vi "Reset Timer.vi"(8 "error in (no error)":errorcluster, 10 "Timer No. (0: All timer number )":string="0", 11 "VISA resource name":refnum<visa-resource-name>) -> (0 "error out":errorcluster, 3 "VISA resource name out":refnum<visa-resource-name>)   [LabVIEW 2020, in "Yokogawa GX Series.lvlib"]
doc: "Reset the relative time timer."
uses:
  <instrlib>/Yokogawa GX Series/Yokogawa GX Series.lvlib
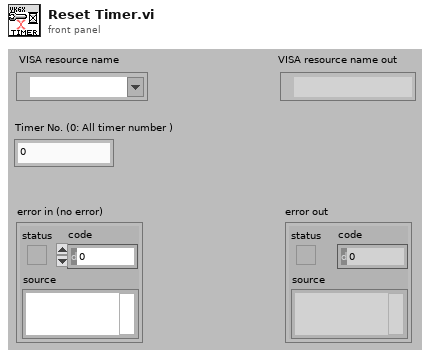
[diagram p1: front panel]
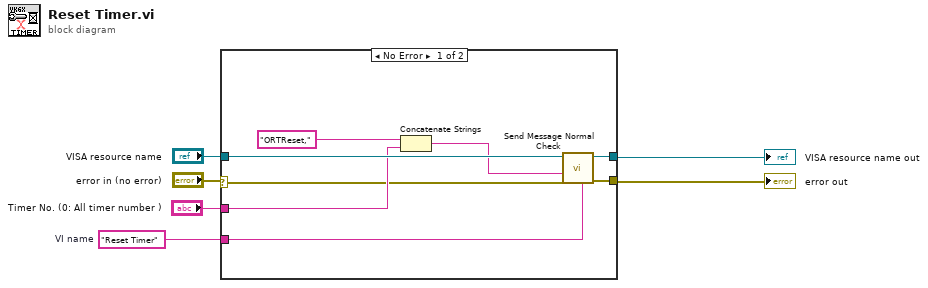
[diagram p0: block diagram]
diagram:
  w3 = "Reset Timer"  # VI name
  n1 = case shown="No Error" "error in (no error)" {
    selector: "error in (no error)" -> [w7 w15]
    tunnel: "VISA resource name" -> [w11 w16]
    tunnel: [w14 w16] -> w5
    tunnel: [w13 w15] -> w4
    tunnel: w3 -> [w12 _]
    tunnel: "Timer No. (0: All timer number )" -> [w9 _]
    frame No Error {
      n2 = Concatenate Strings("ORTReset,", w9) -> (w8:string)
      n3 = call <instrlib>:"Send Message Normal Check.vi"("Source (\"\")"=w12, "error in (no error)"=w7, "Send Message (\"\")"=w8, "VISA resource name"=w11) -> ("error out"=w13:errorcluster, "VISA resource name out"=w14:refnum<visa-resource-name>)  [unwired: 2 in, 4 out]
    }
    frame Error {
    }
  }
  "error out" <- w4
  "VISA resource name out" <- w5
